vi "DSG Generate Waveform.vi"(6 "hardware sync commands queue":refnum<queue>, 7 "measurement configuration":T3={"Input channel"=0, "Full scale range"=10.0, "Input signal"=0, "Analog source resource name"="", "Sine frequency"=1000.0, "Sine amplitude"=5.1, "Triangle frequency"=20.0, "Triangle amplitude"=5.1, "Ramp duration"=10.0, "Ramp amplitude"=5.05, "Ramp type"=0, "Digital capture resource name"="", "Digital capture sample rate"=800000.0, "Digital capture test duration"=10.0} {"Ramp type" items=["Ascending", "Descending"]; "Input signal" items=["Sine", "Triangle", "Ramp"]}, 8 "error in":errorcluster, 11 "meas logic calculated values":T2) -> (0 "error out":errorcluster, 3 "DSG task out":refnum<k21>)   [LabVIEW 2021, in "adc_linearityMeasurement.lvlib"]
uses:
  adc_linearityMeasurement.lvlib
  shared/subVIs/controls/HW Sync Commands.ctl
  Measurement Configuration.ctl
  <vilib>/gRPC/LabVIEW gRPC Library/Shared/grpcId.ctl
  <vilib>/addons/_NISVFA/_Generation/Signal Generation/SV Signal/sv_System Timing Model.ctl
  <vilib>/DAQmx/write.llb/DAQmx Write (Analog Wfm 1Chan NSamp).vi
  <vilib>/DAQmx/write.llb/DAQmx Write (Analog 1D Wfm NChan NSamp).vi
  <vilib>/Analysis/1siggen.llb/Ramp Pattern by Samples.vi
  <vilib>/DAQmx/write.llb/DAQmx Write (Analog 1D DBL 1Chan NSamp).vi
  <vilib>/addons/_NISVFA/_Generation/Signal Generation/SV Sinusoid/SV Sinusoid.lvclass
  C:/Program Files/National Instruments/LabVIEW 2021/vi.lib/addons/_NISVFA/_Generation/Signal Generation/SV Signal/SV Signal.lvclass
  <vilib>/addons/_NISVFA/_Generation/Signal Generation/SV Triangle/SV Triangle.lvclass
  <vilib>/addons/_NISVFA/_Generation/Signal Generation/SV Sinusoid/Configure Sine.vi
  <vilib>/addons/_NISVFA/_Generation/Signal Generation/SV Signal/Write Sample Rate.vi
  <vilib>/addons/_NISVFA/_Generation/Signal Generation/SV Signal/Write System Timing Model.vi
  <vilib>/addons/_NISVFA/_Generation/Signal Generation/SV Signal/Write Ramp Parameters.vi
  <vilib>/DAQmx/miscellaneous.llb/DAQmx Fill In Error Info.vi
  <vilib>/addons/_NISVFA/_Generation/Signal Generation/SV Triangle/Configure Triangle.vi
  <resource>/objmgr/daqmx.rc
  <vilib>/addons/_NISVFA/_Generation/Signal Generation/SV Signal/SV Signal.lvclass
  <vilib>/Analysis/NI_AALBase.lvlib
  <vilib>/gRPC/LabVIEW gRPC Library/grpc-lvsupport-release.lvlib
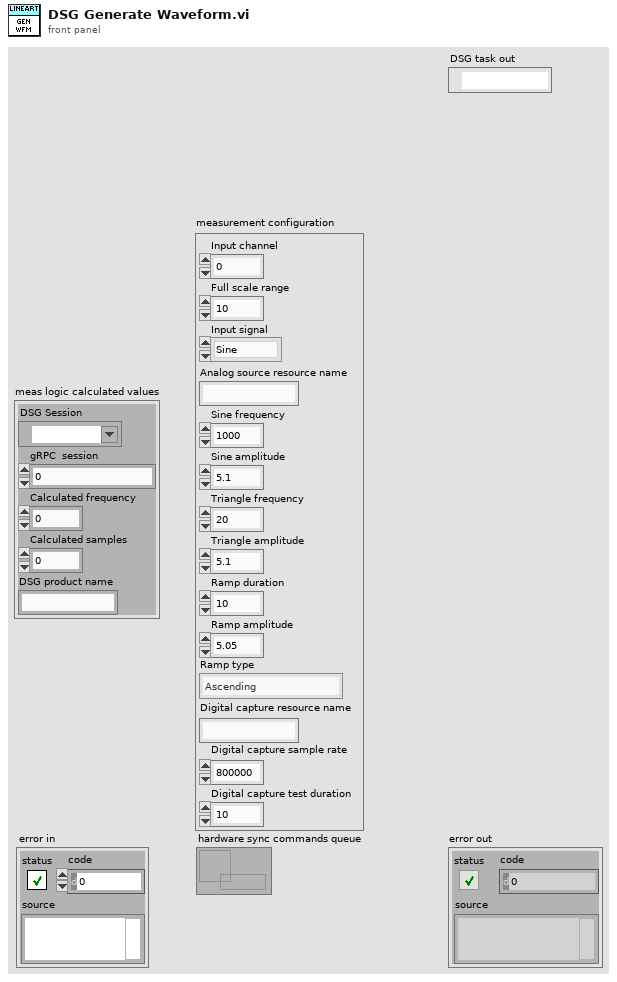
[diagram p1: front panel]
types:
  T1 = typedef "grpc-lvsupport-release.lvlib/grpcId.ctl" = u64
  T2 = cluster{"DSG Session":refnum<k21>, "gRPC  session":T1, "Calculated frequency":dbl, "Calculated samples":u32, "DSG product name":string}
  T3 = typedef "adc_linearityMeasurement.lvlib/Measurement Configuration.ctl" = cluster{"Input channel":i32, "Full scale range":dbl, "Input signal":u16, "Analog source resource name":string, "Sine frequency":dbl, "Sine amplitude":dbl, "Triangle frequency":dbl, "Triangle amplitude":dbl, "Ramp duration":dbl, "Ramp amplitude":dbl, "Ramp type":u16, "Digital capture resource name":string, "Digital capture sample rate":dbl, "Digital capture test duration":dbl}
  T4 = typedef "HW Sync Commands.ctl" = enum16{"NoAction", "GenerationStarted", "AcquisitionCompleted", "GenerationErrored"}
  T5 = cluster{"profile":enum16{"Linear", "Half cosine"}, "durations [s]":cluster{"ramp-up":dbl, "transition":dbl, "ramp-down":dbl}}
  T6 = typedef "SV Signal.lvclass/sv_System Timing Model.ctl" = i64
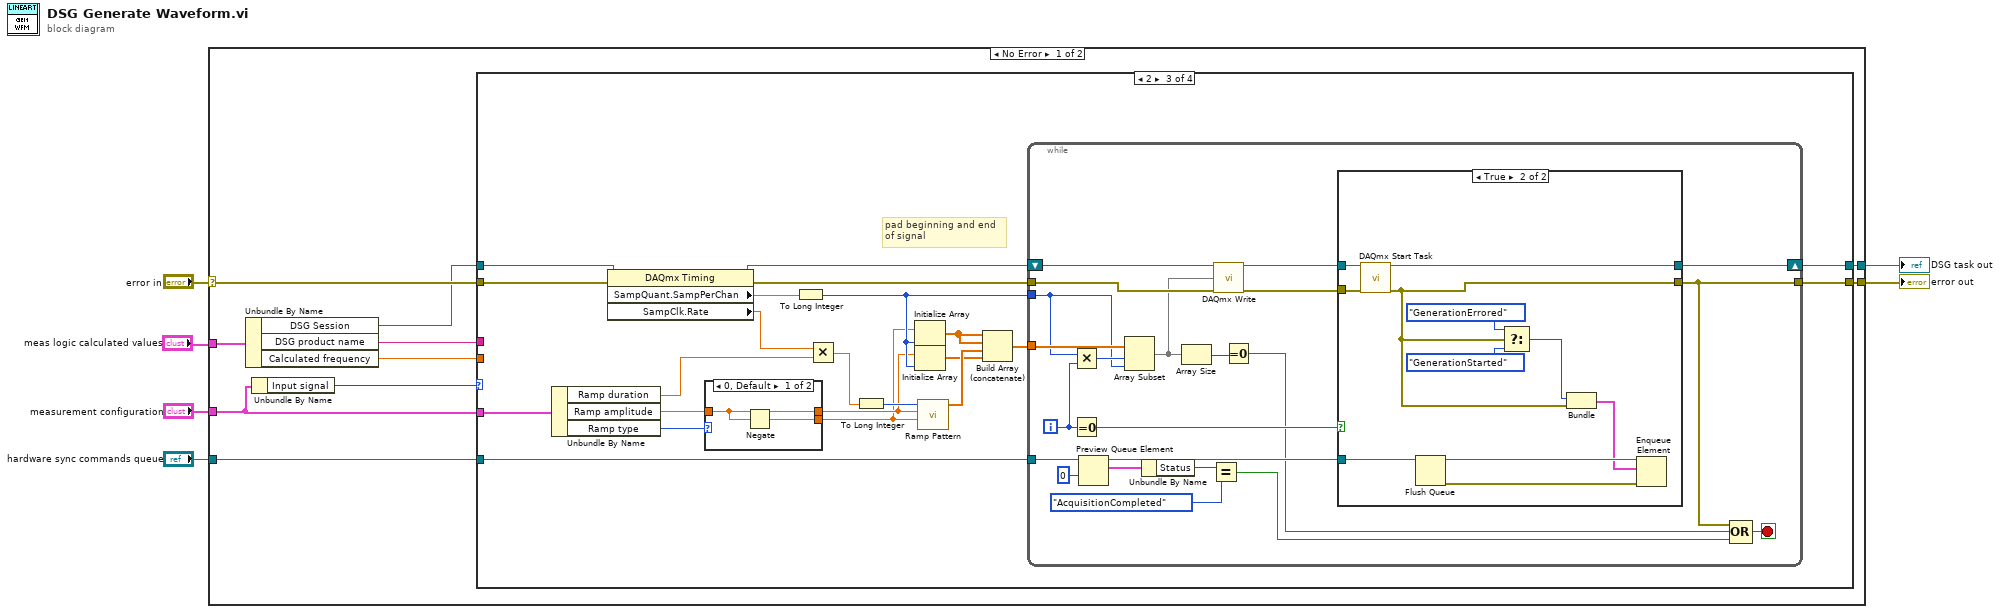
[diagram p0: block diagram]
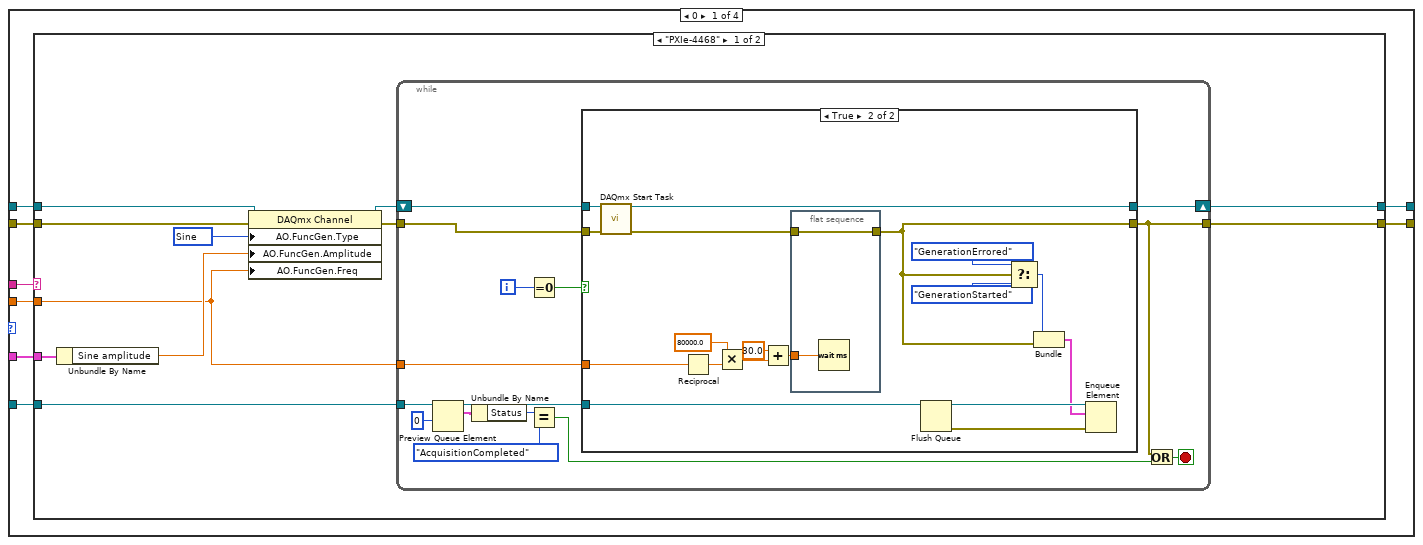
[diagram p2: hidden frame]
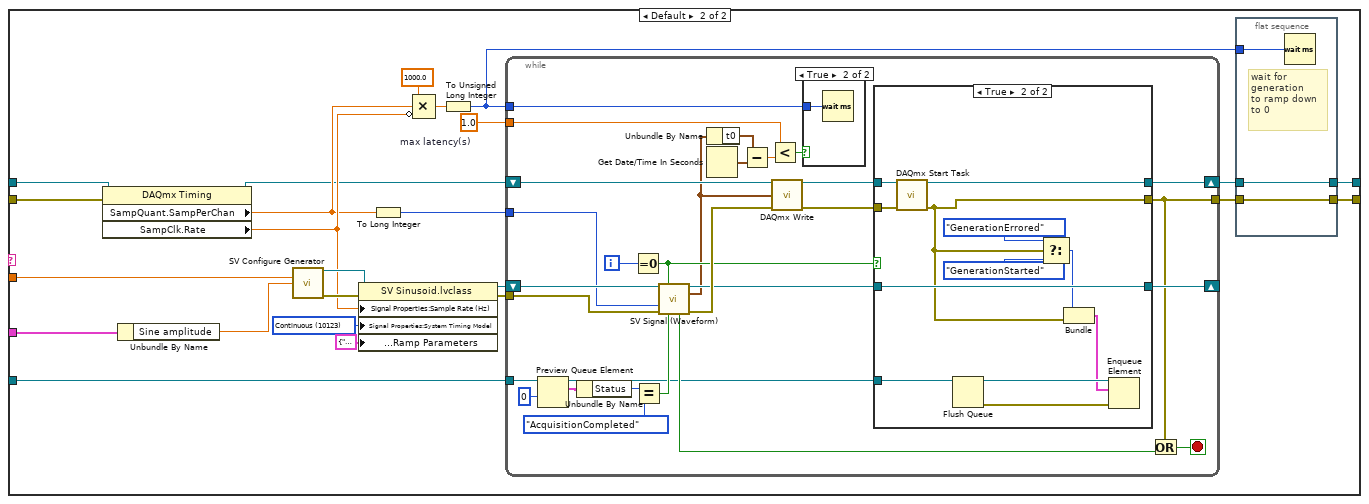
[diagram p4: hidden frame]
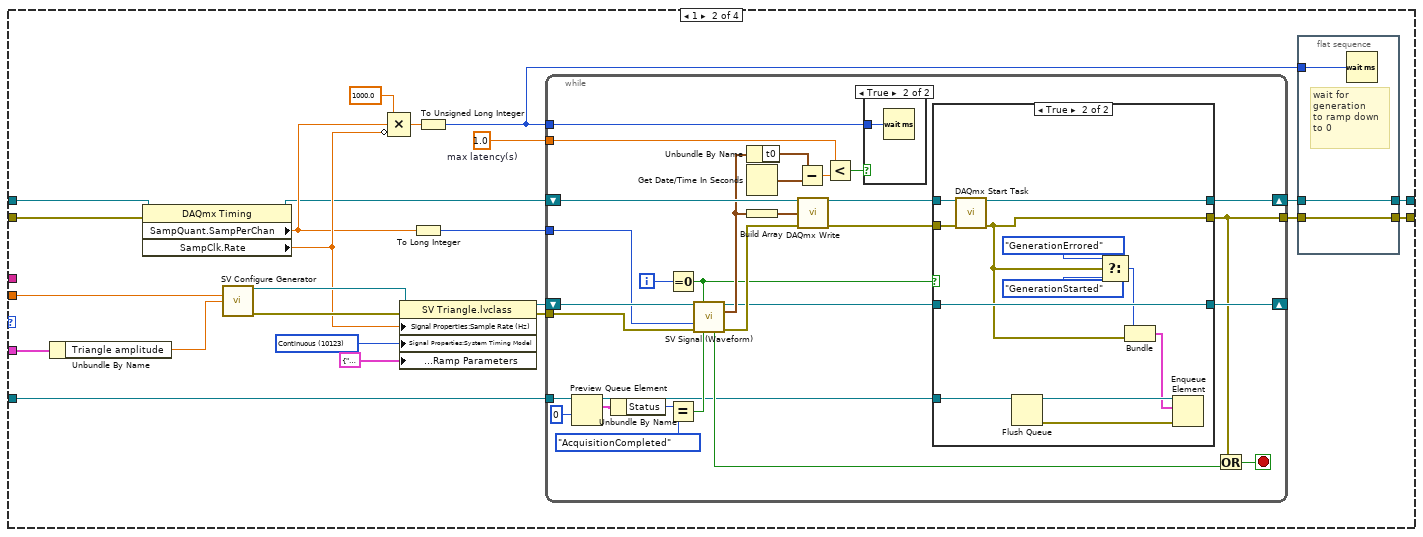
[diagram p7: hidden frame]
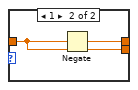
[diagram p10: hidden frame]
diagram:
  n1 = case shown="No Error" "error in" {
    selector: "error in" -> [w16 w281]
    tunnel: [w15 _] -> w5
    tunnel: [w14 w281] -> w4
    tunnel: "hardware sync commands queue" -> [w13 _]
    tunnel: "measurement configuration" -> [w12 _]
    tunnel: "meas logic calculated values" -> [w10 _]
    frame No Error {
      n2 = Unbundle By Name(w10) -> ("DSG Session"=w9:refnum<k21>, "DSG product name"=w8:string, "Calculated frequency"=w7:dbl)
      n3 = Unbundle By Name(w12) -> ("Input signal"=w11:u16)
      n4 = case shown="2" w11 {
        tunnel: w16 -> [w24 w168 w239 w280]
        tunnel: w9 -> [w23 w164 w238 w279]
        tunnel: [w22 w152 w235 w279] -> w15
        tunnel: [w21 w151 w234 w280] -> w14
        tunnel: w13 -> [w20 w149 w233 _]
        tunnel: w12 -> [w19 w147 w231 _]
        tunnel: w8 -> [w18 _ _ _]
        tunnel: w7 -> [w17 w145 _ _]
        frame 0 {
          n5 = case shown="\"PXIe-4468\"" w18 {
            tunnel: w24 -> [w27 w96]
            tunnel: w23 -> [w29 w92]
            tunnel: [w34 w80] -> w22
            tunnel: [w33 w79] -> w21
            tunnel: w20 -> [w35 w77]
            tunnel: w19 -> [w32 w75]
            tunnel: w17 -> [w25 w73]
            frame "PXIe-4468" {
              w26 = 14751 items=["Sine"=14751, "Triangle"=14752, "Square"=14753, "Sawtooth"=14754] ("AO.FuncGen.Type")
              n6 = Unbundle By Name(w32) -> ("Sine amplitude"=w31:dbl)
              n7 = property class="DAQmx Channel"(reference=w29, error in=w27, "AO.FuncGen.Type"=w26, "AO.FuncGen.Amplitude"=w31, "AO.FuncGen.Freq"=w25) -> (reference out=w30:refnum<k21>, error out=w28:errorcluster)
              n8 = while {
                tunnel: w28 -> [w49]
                shift-right: [w43] -> w34
                shift-left: w30 -> [w48]
                tunnel: [w36] -> w33
                tunnel: w35 -> [w40]
                tunnel: w25 -> [w37]
                i -> [w50]
                stop <- w47 stop-if-true
                n9 = Preview Queue Element(queue=w40, timeout in ms (-1)=0) -> (queue out=w44:refnum<queue>, element=w42:cluster{"Status":T4, "Error":errorcluster})  [unwired: 1 in, 2 out]
                n10 = Unbundle By Name(w42) -> ("Status"=w41:T4)
                n11 = Equal To 0?(x=w50) -> (x = 0?=w39:bool)
                n12 = Equal?(x=w41, y=HW_Sync_Commands."AcquisitionCompleted") -> (x = y?=w38:bool)
                n13 = case shown="True" w39 {
                  tunnel: w44 -> [_ w70]
                  tunnel: w48 -> [w52 w68]
                  tunnel: [w52 w54] -> w43
                  tunnel: w49 -> [w51 w67]
                  tunnel: [w51 w56] -> w36
                  tunnel: w37 -> [_ w53]
                  frame False {
                  }
                  frame True {
                    n14 = call <vilib>:"DAQmx Start Task.vi"("task/channels in"=w68, "error in"=w67) -> ("task out"=w54:refnum<k21>, "error out"=w57:errorcluster)  [unwired: 12 in]
                    n15 = Reciprocal(x=w53) -> (1/x=w58:dbl)
                    n16 = Multiply(x=80000.0, y=w58) -> (x*y=w60:dbl)
                    n17 = Add(x=30.0, y=w60) -> (x+y=w55:dbl)
                    n18 = flat-sequence {
                      tunnel: w57 -> [w72]
                      tunnel: [w72] -> w56
                      tunnel: w55 -> [w71]
                      frame #0 {
                        n19 = Wait (ms)(milliseconds to wait=w71) -> ()  [unwired: 1 out]
                      }
                    }
                    n20 = Flush Queue(queue=w70) -> (queue out=w69:refnum<queue>, error out=w66:errorcluster)  [unwired: 1 in, 1 out]
                    n21 = Select(t=HW_Sync_Commands."GenerationErrored" ("element"), s=w56, f=HW_Sync_Commands."GenerationStarted" ("element")) -> (s? t:f=w63:T4)
                    n22 = Bundle("element"=w63, "error out"=w56) -> (w62:cluster{"element":T4, "error out":errorcluster})  [unwired: 1 in]
                    n23 = Enqueue Element(queue=w69, element=w62, error in (no error)=w66) -> ()  [unwired: 1 in, 3 out]
                  }
                }
                n24 = Or(x=w36, y=w38) -> (x .or. y?=w47:bool)
              }
            }
            frame Default {
              w85 = 1.0  # max latency(s)
              w93 = T6 10123 items=["Finite"=10178, "-"=-1, "Continuous"=10123, "-"=-2, "Settled"=110123, "Averaged"=210123, "Discrete Sweep"=310123, "Continuous Sweep"=410123] ("System Timing Model")
              n25 = property class="DAQmx Timing"(reference=w92, error in=w96) -> (reference out=w86:refnum<k21>, "SampQuant.SampPerChan"=w88:dbl, "SampClk.Rate"=w91:dbl)  [unwired: 1 out]
              n26 = Unbundle By Name(w75) -> ("Sine amplitude"=w74:dbl)
              n27 = call-poly <vilib>:"SV Configure Generator.vi"("frequency (Hz)"=w73, "amplitude"=w74) -> ("signal configuration"=w94:refnum<class "SV Sinusoid.lvclass">, "error out"=w95:errorcluster)  [unwired: 12 in]
              n28 = property class="SV Sinusoid.lvclass"(reference=w94, error in=w95, "Signal Properties:Sample Rate (Hz)"=w91, "Signal Properties:System Timing Model"=w93, "Signal Properties:Ramps:Ramp Parameters"=T5 {"profile"=enum."Linear", "durations [s]"={"ramp-up"=0.0, "transition"=0.0, "ramp-down"=0.01}} ("Ramp Parameters:All Elements")) -> (reference out=w90:refnum<class "SV Sinusoid.lvclass">, error out=w89:errorcluster)
              n29 = To Long Integer(number=w88) -> (32bit integer=w87:i32)
              n30 = Compound Arithmetic op=MULTIPLY(1000.0 ("value"), w88, invert w91) -> (w84:dbl)
              n31 = To Unsigned Long Integer(number=w84) -> (unsigned 32bit integer=w78:u32)
              n32 = while {
                shift-right: [w104] -> _
                shift-left: w90 -> [w128]
                tunnel: w89 -> [w125]
                tunnel: w87 -> [w126]
                shift-right: [w107] -> w81
                shift-left: w86 -> [w124]
                tunnel: [w101] -> w82
                tunnel: w85 -> [w117]
                tunnel: w78 -> [w115]
                tunnel: w77 -> [w114]
                i -> [w127]
                stop <- w121 stop-if-true
                n33 = Preview Queue Element(queue=w114, timeout in ms (-1)=0) -> (queue out=w110:refnum<queue>, element=w103:cluster{"Status":T4, "Error":errorcluster})  [unwired: 1 in, 2 out]
                n34 = Unbundle By Name(w103) -> ("Status"=w102:T4)
                n35 = Equal To 0?(x=w127) -> (x = 0?=w109:bool)
                n36 = Equal?(x=w102, y=HW_Sync_Commands."AcquisitionCompleted") -> (x = y?=w111:bool)
                n37 = call-dynamic "SV Signal (Waveform).vi"("signal configuration"=w128, "reset"=w109, "samples"=w126, "error in (no error)"=w125, "stop"=w111) -> ("signal configuration"=w105:refnum<class "SV Sinusoid.lvclass">, "output waveform"=w100:waveform(dbl), "done"=w122:bool, "error out"=w123:errorcluster)  [unwired: 5 in, 2 out]
                n38 = Unbundle By Name(w100) -> ("t0"=w120:timestamp)
                n39 = Get Date/Time In Seconds() -> (seconds since 1Jan1904=w119:timestamp)
                n40 = Subtract(x=w120, y=w119) -> (x-y=w118:dbl)
                n41 = Less?(x=w117, y=w118) -> (x < y?=w116:bool)
                n42 = call-poly <vilib>:"DAQmx Write.vi"("task/channels in"=w124, "data"=w100, "error in"=w123) -> ("task out"=w108:refnum<k21>, "error out"=w106:errorcluster)  [unwired: 10 in, 1 out]
                n43 = case shown="True" w116 {
                  tunnel: w115 -> [_ w144]
                  frame False {
                  }
                  frame True {
                    n44 = Wait (ms)(milliseconds to wait=w144) -> ()  [unwired: 1 out]
                  }
                }
                n45 = case shown="True" w109 {
                  tunnel: w110 -> [_ w143]
                  tunnel: w108 -> [w131 w141]
                  tunnel: [w131 w140] -> w107
                  tunnel: w106 -> [w130 w139]
                  tunnel: [w130 w133] -> w101
                  tunnel: w105 -> [w129 w135]
                  tunnel: [w129 w135] -> w104
                  frame False {
                  }
                  frame True {
                    n46 = call <vilib>:"DAQmx Start Task.vi"("task/channels in"=w141, "error in"=w139) -> ("task out"=w140:refnum<k21>, "error out"=w133:errorcluster)  [unwired: 12 in]
                    n47 = Flush Queue(queue=w143) -> (queue out=w142:refnum<queue>, error out=w138:errorcluster)  [unwired: 1 in, 1 out]
                    n48 = Select(t=HW_Sync_Commands."GenerationErrored" ("element"), s=w133, f=HW_Sync_Commands."GenerationStarted" ("element")) -> (s? t:f=w134:T4)
                    n49 = Bundle("element"=w134, "error out"=w133) -> (w132:cluster{"element":T4, "error out":errorcluster})  [unwired: 1 in]
                    n50 = Enqueue Element(queue=w142, element=w132, error in (no error)=w138) -> ()  [unwired: 1 in, 3 out]
                  }
                }
                n51 = Or(x=w101, y=w122) -> (x .or. y?=w121:bool)
              }
              n52 = flat-sequence {
                tunnel: w82 -> [w98]
                tunnel: w81 -> [w99]
                tunnel: [w99] -> w80
                tunnel: [w98] -> w79
                tunnel: w78 -> [w97]
                frame #0 {
                  # "wait for\ngeneration\nto ramp down\nto 0"
                  n53 = Wait (ms)(milliseconds to wait=w97) -> ()  [unwired: 1 out]
                }
              }
            }
          }
        }
        frame 1 {
          w157 = 1.0  # max latency(s)
          w165 = T6 10123 items=["Finite"=10178, "-"=-1, "Continuous"=10123, "-"=-2, "Settled"=110123, "Averaged"=210123, "Discrete Sweep"=310123, "Continuous Sweep"=410123] ("System Timing Model")
          n54 = Unbundle By Name(w147) -> ("Triangle amplitude"=w146:dbl)
          n55 = property class="DAQmx Timing"(reference=w164, error in=w168) -> (reference out=w158:refnum<k21>, "SampQuant.SampPerChan"=w160:dbl, "SampClk.Rate"=w163:dbl)  [unwired: 1 out]
          n56 = call-poly <vilib>:"SV Configure Generator.vi"("frequency (Hz)"=w145, "amplitude"=w146) -> ("signal configuration"=w166:refnum<class "SV Triangle.lvclass">, "error out"=w167:errorcluster)  [unwired: 12 in]
          n57 = Compound Arithmetic op=MULTIPLY(1000.0 ("value"), w160, invert w163) -> (w156:dbl)
          n58 = property class="SV Triangle.lvclass"(reference=w166, error in=w167, "Signal Properties:Sample Rate (Hz)"=w163, "Signal Properties:System Timing Model"=w165, "Signal Properties:Ramps:Ramp Parameters"=T5 {"profile"=enum."Linear", "durations [s]"={"ramp-up"=0.0, "transition"=0.0, "ramp-down"=0.01}} ("Ramp Parameters:All Elements")) -> (reference out=w162:refnum<class "SV Triangle.lvclass">, error out=w161:errorcluster)
          n59 = To Long Integer(number=w160) -> (32bit integer=w159:i32)
          n60 = To Unsigned Long Integer(number=w156) -> (unsigned 32bit integer=w150:u32)
          n61 = while {
            shift-right: [w175] -> _
            shift-left: w162 -> [w201]
            tunnel: w161 -> [w198]
            tunnel: w159 -> [w199]
            shift-right: [w178] -> w153
            shift-left: w158 -> [w197]
            tunnel: [w172] -> w154
            tunnel: w157 -> [w188]
            tunnel: w150 -> [w186]
            tunnel: w149 -> [w185]
            i -> [w200]
            stop <- w193 stop-if-true
            n62 = Preview Queue Element(queue=w185, timeout in ms (-1)=0) -> (queue out=w181:refnum<queue>, element=w174:cluster{"Status":T4, "Error":errorcluster})  [unwired: 1 in, 2 out]
            n63 = Unbundle By Name(w174) -> ("Status"=w173:T4)
            n64 = Equal To 0?(x=w200) -> (x = 0?=w180:bool)
            n65 = Equal?(x=w173, y=HW_Sync_Commands."AcquisitionCompleted") -> (x = y?=w182:bool)
            n66 = call-dynamic "SV Signal (Waveform).vi"("signal configuration"=w201, "reset"=w180, "samples"=w199, "error in (no error)"=w198, "stop"=w182) -> ("signal configuration"=w176:refnum<class "SV Triangle.lvclass">, "output waveform"=w192:waveform(dbl), "done"=w194:bool, "error out"=w195:errorcluster)  [unwired: 5 in, 2 out]
            n67 = Unbundle By Name(w192) -> ("t0"=w191:timestamp)
            n68 = Get Date/Time In Seconds() -> (seconds since 1Jan1904=w190:timestamp)
            n69 = Build Array(w192) -> (w196:waveform(dbl)[])
            n70 = Subtract(x=w191, y=w190) -> (x-y=w189:dbl)
            n71 = call-poly <vilib>:"DAQmx Write.vi"("task/channels in"=w197, "data"=w196, "error in"=w195) -> ("task out"=w179:refnum<k21>, "error out"=w177:errorcluster)  [unwired: 10 in, 1 out]
            n72 = Less?(x=w188, y=w189) -> (x < y?=w187:bool)
            n73 = case shown="True" w187 {
              tunnel: w186 -> [_ w217]
              frame False {
              }
              frame True {
                n74 = Wait (ms)(milliseconds to wait=w217) -> ()  [unwired: 1 out]
              }
            }
            n75 = case shown="True" w180 {
              tunnel: w181 -> [_ w216]
              tunnel: w179 -> [w204 w214]
              tunnel: [w204 w213] -> w178
              tunnel: w177 -> [w203 w212]
              tunnel: [w203 w206] -> w172
              tunnel: w176 -> [w202 w208]
              tunnel: [w202 w208] -> w175
              frame False {
              }
              frame True {
                n76 = call <vilib>:"DAQmx Start Task.vi"("task/channels in"=w214, "error in"=w212) -> ("task out"=w213:refnum<k21>, "error out"=w206:errorcluster)  [unwired: 12 in]
                n77 = Flush Queue(queue=w216) -> (queue out=w215:refnum<queue>, error out=w211:errorcluster)  [unwired: 1 in, 1 out]
                n78 = Select(t=HW_Sync_Commands."GenerationErrored" ("element"), s=w206, f=HW_Sync_Commands."GenerationStarted" ("element")) -> (s? t:f=w207:T4)
                n79 = Bundle("element"=w207, "error out"=w206) -> (w205:cluster{"element":T4, "error out":errorcluster})  [unwired: 1 in]
                n80 = Enqueue Element(queue=w215, element=w205, error in (no error)=w211) -> ()  [unwired: 1 in, 3 out]
              }
            }
            n81 = Or(x=w172, y=w194) -> (x .or. y?=w193:bool)
          }
          n82 = flat-sequence {
            tunnel: w154 -> [w170]
            tunnel: w153 -> [w171]
            tunnel: [w171] -> w152
            tunnel: [w170] -> w151
            tunnel: w150 -> [w169]
            frame #0 {
              # "wait for\ngeneration\nto ramp down\nto 0"
              n83 = Wait (ms)(milliseconds to wait=w169) -> ()  [unwired: 1 out]
            }
          }
        }
        frame 2 {
          # "pad beginning and end\nof signal"
          n84 = Unbundle By Name(w231) -> ("Ramp duration"=w230:dbl, "Ramp amplitude"=w220:dbl, "Ramp type"=w221:u16)
          n85 = property class="DAQmx Timing"(reference=w238, error in=w239) -> (reference out=w236:refnum<k21>, error out=w224:errorcluster, "SampQuant.SampPerChan"=w237:dbl, "SampClk.Rate"=w229:dbl)
          n86 = case shown="0, Default" w221 {
            tunnel: w220 -> [w241 w243]
            tunnel: [w241 w242] -> w219
            tunnel: [w240 w243] -> w218
            frame 0, Default {
              n87 = Negate(x=w241) -> (-x=w240:dbl)
            }
            frame 1 {
              n88 = Negate(x=w243) -> (-x=w242:dbl)
            }
          }
          n89 = To Long Integer(number=w237) -> (32bit integer=w222:i32)
          n90 = Multiply(x=w229, y=w230) -> (x*y=w228:dbl)
          n91 = To Long Integer(number=w228) -> (32bit integer=w232:i32)
          n92 = Initialize Array(w218, w222) -> (w226:dbl[])
          n93 = Initialize Array(w219, w222) -> (w225:dbl[])
          n94 = call-poly <vilib>:"Ramp Pattern.vi"("start"=w218, "end"=w219, "samples"=w232) -> ("Ramp Pattern"=w227:dbl[])  [unwired: 7 in, 1 out]
          n95 = Build Array (concatenate)(w226, w226, w227, w225) -> (w223:dbl[])
          n96 = while {
            shift-right: [w257] -> w235
            shift-left: w236 -> [w265]
            tunnel: [w244] -> w234
            tunnel: w233 -> [w263]
            tunnel: w224 -> [w256]
            tunnel: w223 -> [w254]
            tunnel: w222 -> [w251]
            i -> [w253]
            stop <- w264 stop-if-true
            n97 = Multiply(x=w251, y=w253) -> (x*y=w252:i32)
            n98 = Equal To 0?(x=w253) -> (x = 0?=w259:bool)
            n99 = Preview Queue Element(queue=w263, timeout in ms (-1)=0) -> (queue out=w260:refnum<queue>, element=w246:cluster{"Status":T4, "Error":errorcluster})  [unwired: 1 in, 2 out]
            n100 = Array Subset(array=w254, index=w252, length=w251) -> (w249:dbl[])
            n101 = Unbundle By Name(w246) -> ("Status"=w245:T4)
            n102 = Array Size(array=w249) -> (size(s)=w248:i32)
            n103 = Equal?(x=w245, y=HW_Sync_Commands."AcquisitionCompleted") -> (x = y?=w255:bool)
            n104 = call-poly <vilib>:"DAQmx Write.vi"("task/channels in"=w265, "data"=w249, "error in"=w256) -> ("task out"=w258:refnum<k21>, "error out"=w250:errorcluster)  [unwired: 10 in, 1 out]
            n105 = Equal To 0?(x=w248) -> (x = 0?=w247:bool)
            n106 = case shown="True" w259 {
              tunnel: w260 -> [_ w278]
              tunnel: w258 -> [w267 w276]
              tunnel: [w267 w275] -> w257
              tunnel: w250 -> [w266 w274]
              tunnel: [w266 w268] -> w244
              frame False {
              }
              frame True {
                n107 = call <vilib>:"DAQmx Start Task.vi"("task/channels in"=w276, "error in"=w274) -> ("task out"=w275:refnum<k21>, "error out"=w268:errorcluster)  [unwired: 12 in]
                n108 = Flush Queue(queue=w278) -> (queue out=w277:refnum<queue>, error out=w273:errorcluster)  [unwired: 1 in, 1 out]
                n109 = Select(t=HW_Sync_Commands."GenerationErrored" ("element"), s=w268, f=HW_Sync_Commands."GenerationStarted" ("element")) -> (s? t:f=w270:T4)
                n110 = Bundle("element"=w270, "error out"=w268) -> (w269:cluster{"element":T4, "error out":errorcluster})  [unwired: 1 in]
                n111 = Enqueue Element(queue=w277, element=w269, error in (no error)=w273) -> ()  [unwired: 1 in, 3 out]
              }
            }
            n112 = Compound Arithmetic op=OR(w244, w247, w255) -> (w264:bool)
          }
        }
        frame Default {
        }
      }
    }
    frame Error {
    }
  }
  "DSG task out" <- w5
  "error out" <- w4
